vi "获取URL下载链接.vi"(8 "error in (no error)":errorcluster) -> (0 "error out":errorcluster, 3 "String/Binary data":string caption="URL")   [LabVIEW 2016, in "数据传输系统-06.lvlib" / "update.lvlib" / "http client.lvclass"]
uses:
  http client.lvclass
  <vilib>/registry/registry.llb/Registry RtKey.ctl
  <vilib>/registry/registry.llb/Read Registry Value Simple STR.vi
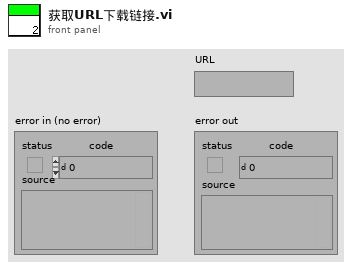
[diagram p1: front panel]
types:
  T1 = typedef "Registry RtKey.ctl" = enum32{"HKEY_CLASSES_ROOT", "HKEY_CURRENT_USER", "HKEY_LOCAL_MACHINE", "HKEY_USERS", "HKEY_PERFORMANCE_DATA", "HKEY_CURRENT_CONFIG", "HKEY_DYN_DATA"}
  T2 = typedef "Registry refnum.ctl" = refnum<k1>
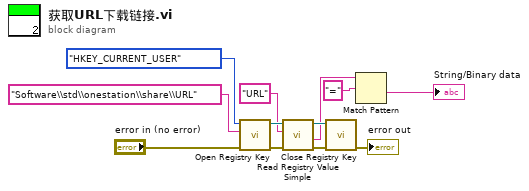
[diagram p0: block diagram]
diagram:
  n1 = call <vilib>:"Open Registry Key.vi"("error in (no error)"="error in (no error)", "subkey"="Software\\std\\onestation\\share\\URL", "root key (HKEY_LOCAL_MACHINE)"=Registry_RtKey."HKEY_CURRENT_USER") -> ("error out"=w11:errorcluster, "refnum out"=w12:T2)  [unwired: 7 in]
  n2 = call-poly <vilib>:"Read Registry Value Simple.vi"("error in (no error)"=w11, "value"="URL", "refnum"=w12) -> ("error out"=w7:errorcluster, "String/Binary data"=w5:string, "refnum out"=w8:T2)  [unwired: 3 in, 1 out]
  n3 = call <vilib>:"Close Registry Key.vi"("error in (no error)"=w7, "refnum"=w8) -> ("error out"=→"error out":errorcluster)  [unwired: 5 in]
  n4 = Match Pattern(string=w5, regular expression="=" ("正则表达式")) -> (after substring=→"String/Binary data":string)  [unwired: 1 in, 3 out]
